vi "Better ReadLEDState.vi"(0 "Front?":bool, 1 "State":string, 5 "LEDs":T1) -> (6 "RED":bool, 7 "GREEN":bool, 8 "BLUE":bool)   [LabVIEW 2016]
uses:
  Common Code/LED Dashboard.ctl
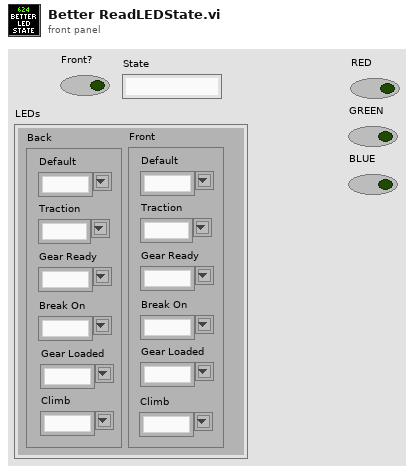
[diagram p1: front panel]
types:
  T1 = typedef "LED Dashboard.ctl" = cluster{"Back":cluster{"Traction":string, "Gear Ready":string, "Default":string, "Break On":string, "Gear Loaded":string, "Climb":string}, "Front":cluster{"Traction":string, "Gear Ready":string, "Default":string, "Break On":string, "Gear Loaded":string, "Climb":string}}
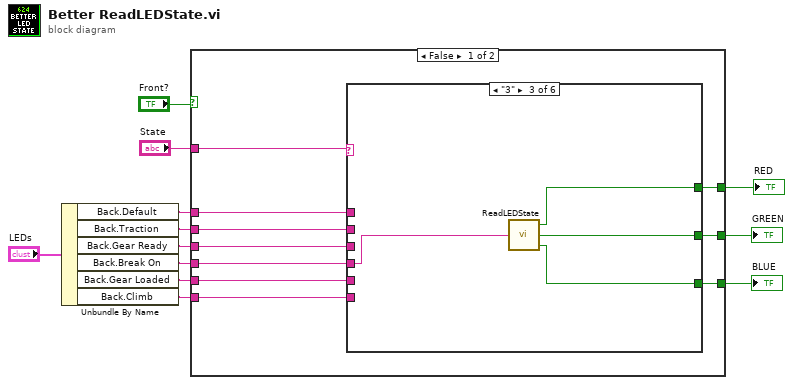
[diagram p0: block diagram]
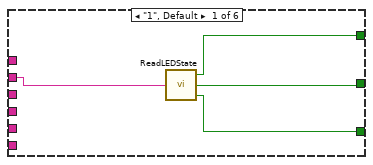
[diagram p2: hidden frame]
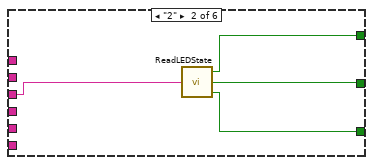
[diagram p3: hidden frame]
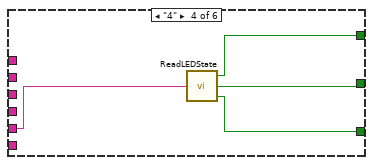
[diagram p4: hidden frame]
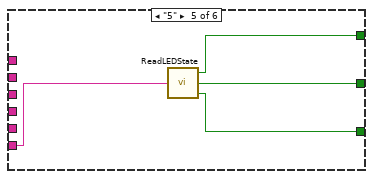
[diagram p5: hidden frame]
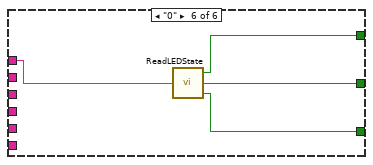
[diagram p6: hidden frame]
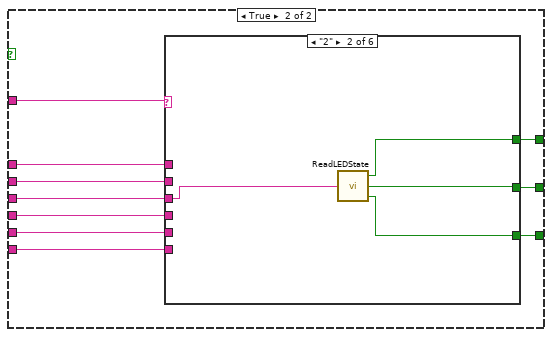
[diagram p7: hidden frame]
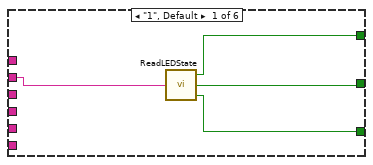
[diagram p8: hidden frame]
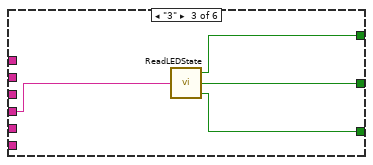
[diagram p9: hidden frame]
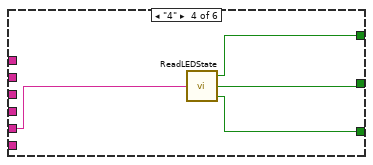
[diagram p10: hidden frame]
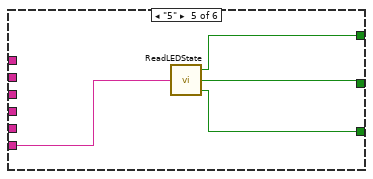
[diagram p11: hidden frame]
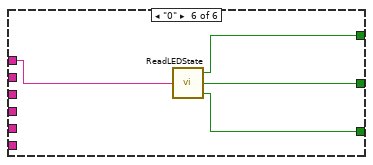
[diagram p12: hidden frame]
diagram:
  n1 = Unbundle By Name("LEDs") -> ("Back.Default"=w6:string, "Back.Traction"=w5:string, "Back.Gear Ready"=w4:string, "Back.Break On"=w3:string, "Back.Gear Loaded"=w2:string, "Back.Climb"=w1:string)
  n2 = case shown="False" "Front?" {
    tunnel: "State" -> [w19 w56]
    tunnel: [w22 w55] -> w10
    tunnel: [w21 w54] -> w9
    tunnel: [w20 w53] -> w8
    tunnel: w6 -> [w18 w52]
    tunnel: w5 -> [w17 w51]
    tunnel: w4 -> [w16 w50]
    tunnel: w3 -> [w15 w49]
    tunnel: w2 -> [w14 w48]
    tunnel: w1 -> [w13 w47]
    frame False {
      n3 = case shown="\"3\"" w19 {
        tunnel: w18 -> [_ _ _ _ _ w43]
        tunnel: w17 -> [w23 _ _ _ _ _]
        tunnel: w16 -> [_ w27 _ _ _ _]
        tunnel: w15 -> [_ _ w31 _ _ _]
        tunnel: w14 -> [_ _ _ w35 _ _]
        tunnel: [w25 w29 w33 w37 w41 w46] -> w22
        tunnel: [w26 w30 w34 w38 w40 w45] -> w21
        tunnel: [w24 w28 w32 w36 w39 w44] -> w20
        tunnel: w13 -> [_ _ _ _ w42 _]
        frame "1", Default {
          n4 = call "ReadLEDState.vi"("State"=w23) -> ("BLUE"=w24:bool, "GREEN"=w26:bool, "RED"=w25:bool)  [unwired: 2 in]
        }
        frame "2" {
          n5 = call "ReadLEDState.vi"("State"=w27) -> ("BLUE"=w28:bool, "GREEN"=w30:bool, "RED"=w29:bool)  [unwired: 2 in]
        }
        frame "3" {
          n6 = call "ReadLEDState.vi"("State"=w31) -> ("BLUE"=w32:bool, "GREEN"=w34:bool, "RED"=w33:bool)  [unwired: 2 in]
        }
        frame "4" {
          n7 = call "ReadLEDState.vi"("State"=w35) -> ("BLUE"=w36:bool, "GREEN"=w38:bool, "RED"=w37:bool)  [unwired: 2 in]
        }
        frame "5" {
          n8 = call "ReadLEDState.vi"("State"=w42) -> ("BLUE"=w39:bool, "GREEN"=w40:bool, "RED"=w41:bool)  [unwired: 2 in]
        }
        frame "0" {
          n9 = call "ReadLEDState.vi"("State"=w43) -> ("BLUE"=w44:bool, "GREEN"=w45:bool, "RED"=w46:bool)  [unwired: 2 in]
        }
      }
    }
    frame True {
      n10 = case shown="\"2\"" w56 {
        tunnel: w52 -> [_ _ _ _ _ w77]
        tunnel: w51 -> [w57 _ _ _ _ _]
        tunnel: w50 -> [_ w61 _ _ _ _]
        tunnel: w49 -> [_ _ w65 _ _ _]
        tunnel: w48 -> [_ _ _ w69 _ _]
        tunnel: [w59 w63 w67 w71 w75 w80] -> w55
        tunnel: [w60 w64 w68 w72 w76 w79] -> w54
        tunnel: [w58 w62 w66 w70 w74 w78] -> w53
        tunnel: w47 -> [_ _ _ _ w73 _]
        frame "1", Default {
          n11 = call "ReadLEDState.vi"("State"=w57) -> ("BLUE"=w58:bool, "GREEN"=w60:bool, "RED"=w59:bool)  [unwired: 2 in]
        }
        frame "2" {
          n12 = call "ReadLEDState.vi"("State"=w61) -> ("BLUE"=w62:bool, "GREEN"=w64:bool, "RED"=w63:bool)  [unwired: 2 in]
        }
        frame "3" {
          n13 = call "ReadLEDState.vi"("State"=w65) -> ("BLUE"=w66:bool, "GREEN"=w68:bool, "RED"=w67:bool)  [unwired: 2 in]
        }
        frame "4" {
          n14 = call "ReadLEDState.vi"("State"=w69) -> ("BLUE"=w70:bool, "GREEN"=w72:bool, "RED"=w71:bool)  [unwired: 2 in]
        }
        frame "5" {
          n15 = call "ReadLEDState.vi"("State"=w73) -> ("BLUE"=w74:bool, "GREEN"=w76:bool, "RED"=w75:bool)  [unwired: 2 in]
        }
        frame "0" {
          n16 = call "ReadLEDState.vi"("State"=w77) -> ("BLUE"=w78:bool, "GREEN"=w79:bool, "RED"=w80:bool)  [unwired: 2 in]
        }
      }
    }
  }
  "RED" <- w10
  "GREEN" <- w9
  "BLUE" <- w8
